vi "Configure PointScan.vi"(0 "AODAcq in":refnum<class "AODAcq.lvclass">, 1 "Save":bool, 5 "Points":i32[][](array[numeric]), 7 "GridSize":u32, 9 "Reps":u32, 11 "error in (no error)":errorcluster, 12 "Motion Points":u32, 14 "Motion Increment":u32) -> (4 "AODAcq out":refnum<class "AODAcq.lvclass">, 15 "error out":errorcluster)   [LabVIEW 2011, in "AODAcq.lvclass"]
uses:
  AODAcq.lvclass
  AODAcq.lvclass/AODAcq.ctl
  <vilib>/Utility/error.llb/Error Cluster From Error Code.vi
  Program Files/National Instruments/LabVIEW 2011/Targets/NI/FPGA/StockFPGA_IntfPrivate/ScriptTemplates/StockFPGA_PlugInRead32.vi
  <vilib>/rvi/errors/niLvFpgaAdjustHostInterfaceError.vi
  <vilib>/rvi/interface/nirviReadWriteControl/nirviReadWriteControl.xnode
  FPGA_Control/AODRef.ctl
  FPGA Bitfiles/Acquisition_FPGATarget_AODControl(FPGA)_C1C38267.lvbitx
  FPGA_Control/AOD Control (FPGA).vi
  HDF5Tools/LabView/HDF5Tools.lvlib
  NiFpgaLv.dll
  <vilib>/FPGAPlugInAG/PXIe-7965R/niLvFpga_Read32_PXIe-7965R.vi
  <vilib>/rvi/interface/nirviReadWriteControl/niFpgaRWControlAccessTimeoutTemplate.vi
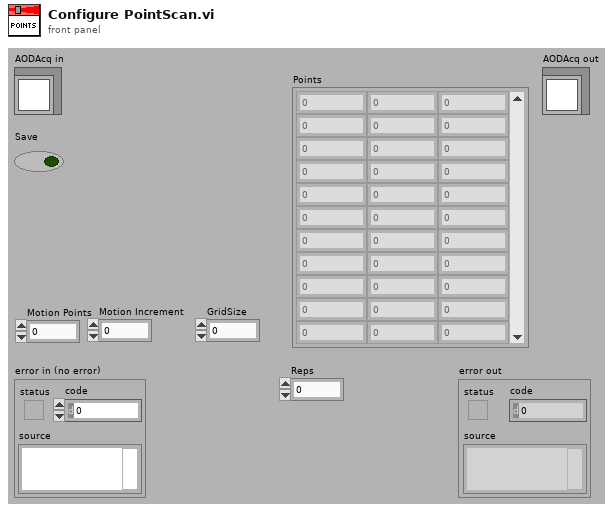
[diagram p1: front panel]
types:
  T1 = typedef "AODRef.ctl" = refnum<k20>
  T2 = cluster{"file handle out":i32, "ImData":i32, "TemporalData":i32, "MotionData":i32}
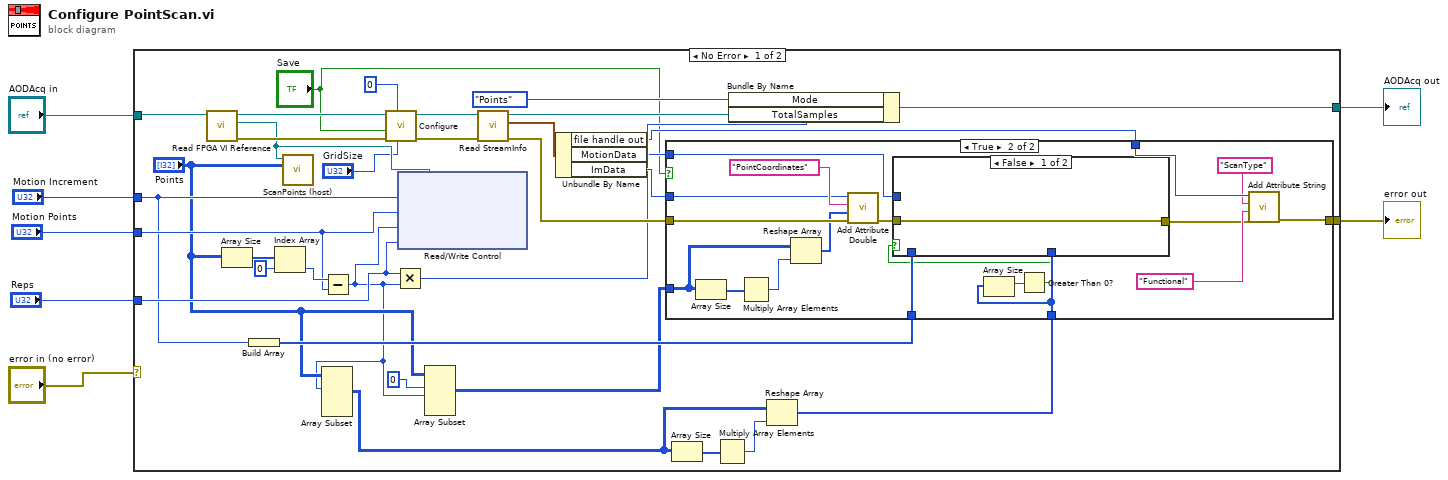
[diagram p0: block diagram]
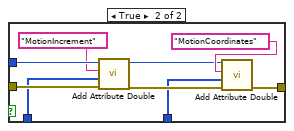
[diagram p3: hidden frame]
diagram:
  n1 = case shown="No Error" "error in (no error)" {
    selector: "error in (no error)" -> [_ w72]
    tunnel: [w32 w72] -> w6
    tunnel: [w28 w71] -> w4
    tunnel: "AODAcq in" -> [w40 w71]
    tunnel: "Motion Increment" -> [w20 _]
    tunnel: "Motion Points" -> [w21 _]
    tunnel: "Reps" -> [w23 _]
    frame No Error {
      n2 = call-dynamic "Read FPGA VI Reference.vi"("AODAcq in"=w40) -> ("error out"=w37:errorcluster, "FPGA VI Reference"=w25:T1, "AODAcq out"=w39:refnum<class "AODAcq.lvclass">)  [unwired: 8 in]
      n3 = Array Size(array="Points") -> (size(s)=w31:i32[])
      n4 = Build Array(w20) -> (w18:u32[])
      n5 = Index Array(array=w31, index=0) -> (element=w24:i32)
      n6 = call "ScanPoints (host).vi"("Points"="Points", "FPGA VI Reference Out"=w25) -> ()  [unwired: 10 in]
      n7 = Subtract(x=w24, y=w21) -> (x-y=w14:u32)
      n8 = Array Subset(array="Points", index (row)=w14) -> (w11:i32[][])  [unwired: 3 in]
      n9 = call-dynamic "Configure.vi"("GridSize"="GridSize", "Mode"=u32 0, "error in (no error)"=w37, "Save"="Save", "AODAcq in"=w39) -> ("error out"=w36:errorcluster, "AODAcq out"=w38:refnum<class "AODAcq.lvclass">)  [unwired: 5 in]
      n10 = Multiply(x=w23, y=w14) -> (x*y=w27:u32)
      n11 = xnode "Read/Write Control"("FPGA VI Reference In"=w25, "Scan.Motion Increment"=w20, "Scan.NumMotionPoints"=w21, "Scan.NumPoints"=w14, "Scan.NumReps"=w23) -> ()  [unwired: 1 in, 2 out]
      n12 = Array Subset(array="Points", index (row)=0 ("index"), length (row)=w14) -> (w16:i32[][])  [unwired: 2 in]
      n13 = call-dynamic "Read StreamInfo.vi"("error in (no error)"=w36, "AODAcq in"=w38) -> ("error out"=w33:errorcluster, "StreamInfo"=w35:T2, "AODAcq out"=w29:refnum<class "AODAcq.lvclass">)  [unwired: 7 in]
      n14 = Unbundle By Name(w35) -> ("file handle out"=w9:i32, "MotionData"=w19:i32, "ImData"=w34:i32)
      n15 = Array Size(array=w11) -> (size(s)=w12:i32[])
      n16 = Multiply Array Elements(1:w12) -> (0:w13:i32)
      n17 = Bundle By Name(cluster=w29, "Mode"=enum16{"Idle", "Points", "Volume"}."Points", "TotalSamples"=w27) -> (w28:refnum<class "AODAcq.lvclass">)
      n18 = Reshape Array(w11, w13) -> (w10:i32[])
      n19 = case shown="True" "Save" {
        tunnel: w34 -> [_ w56]
        tunnel: w16 -> [_ w58]
        tunnel: w33 -> [w42 w55]
        tunnel: [w42 w50] -> w32
        tunnel: w19 -> [_ w53]
        tunnel: w18 -> [_ w51]
        tunnel: w10 -> [_ w48]
        tunnel: w9 -> [_ w49]
        frame False {
        }
        frame True {
          n20 = Array Size(array=w58) -> (size(s)=w59:i32[])
          n21 = Multiply Array Elements(1:w59) -> (0:w60:i32)
          n22 = Reshape Array(w58, w60) -> (w54:i32[])
          n23 = call "Add Attribute Double.vi"("error in (no error)"=w55, "data"=w54, "Attribute name"="PointCoordinates", "loc_id"=w56) -> ("error out"=w52:errorcluster)  [unwired: 6 in, 1 out]
          n24 = Array Size(array=w48) -> (size(s)=w47:i32)
          n25 = Greater Than 0?(x=w47) -> (x > 0?=w46:bool)
          n26 = case shown="False" w46 {
            tunnel: w53 -> [_ w70]
            tunnel: w52 -> [w61 w69]
            tunnel: w51 -> [_ w68]
            tunnel: w48 -> [_ w64]
            tunnel: [w61 w62] -> w43
            frame False {
            }
            frame True {
              n27 = call "Add Attribute Double.vi"("error in (no error)"=w69, "data"=w68, "Attribute name"="MotionIncrement", "loc_id"=w70) -> ("error out"=w66:errorcluster, "loc_id_out"=w63:i32)  [unwired: 6 in]
              n28 = call "Add Attribute Double.vi"("error in (no error)"=w66, "data"=w64, "Attribute name"="MotionCoordinates", "loc_id"=w63) -> ("error out"=w62:errorcluster)  [unwired: 6 in, 1 out]
            }
          }
          n29 = call "Add Attribute String.vi"("error in (no error)"=w43, "Attribute data"="Functional", "Attribute name"="ScanType", "loc_id"=w49) -> ("error out"=w50:errorcluster)  [unwired: 6 in, 1 out]
        }
      }
    }
    frame Error {
    }
  }
  "error out" <- w6
  "AODAcq out" <- w4
